vi "GetElements(Multiple).vi"(7 "Qualified Name":string, 8 "error in (no error)":errorcluster, 10 "keys":string[](array[string]), 11 "SMOConfigManagerCollection in":refnum<class "ConfigManagerCollection.lvclass">) -> (0 "error out":errorcluster, 1 "Found":bool[](array[boolean]), 2 "Values":string[](array[string]), 3 "SMOConfigManagerCollection out":refnum<class "ConfigManagerCollection.lvclass">)   [LabVIEW 2013, in "SMOConfig.lvlib" / "ConfigManagerCollection.lvclass"]
uses:
  ConfigManagerCollection.lvclass
  Manager/ConfigManager.lvclass
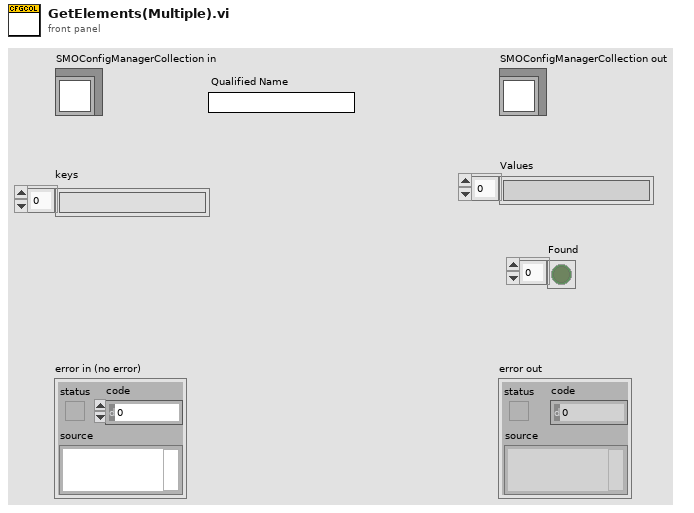
[diagram p1: front panel]
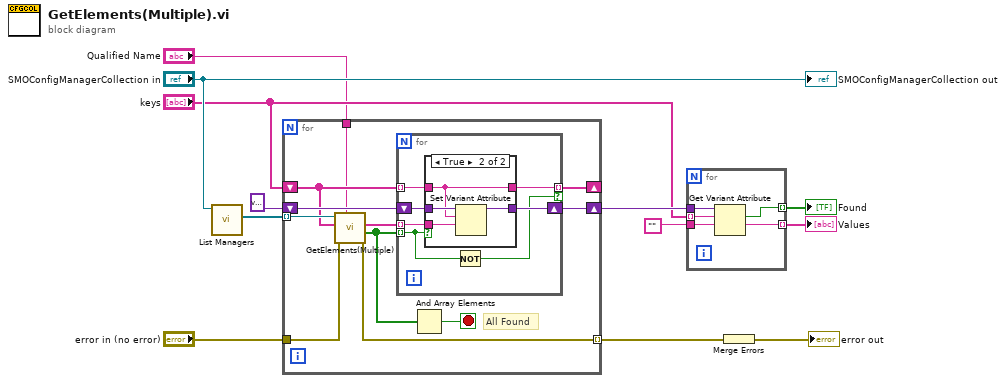
[diagram p0: block diagram]
diagram:
  n1 = call-dynamic "List Managers.vi"("SMOConfigManagerCollection in"="SMOConfigManagerCollection in") -> ("List"=w12:refnum<class "ConfigManager.lvclass">[])  [unwired: 9 in, 1 out]
  n2 = for {
    tunnel: w12 -> [w23] mode=indexing
    tunnel: "error in (no error)" -> [w21]
    tunnel: [w20] -> w11 mode=indexing
    shift-right: [w17] -> w6
    shift-left: variant ("variant") -> [w18]
    shift-right: [w14] -> _
    shift-left: "keys" -> [w15]
    tunnel: "Qualified Name" -> [w13]
    stop <- w22 stop-if-true
    # "All Found"
    n3 = call-dynamic "GetElements(Multiple).vi"("Qualified Name"=w13, "error in (no error)"=w21, "keys"=w15, "SMOConfigManager in"=w23) -> ("error out"=w20:errorcluster, "Found"=w19:bool[], "Values"=w16:string[])  [unwired: 4 in, 1 out]
    n4 = for {
      tunnel: w19 -> [w25] mode=indexing
      shift-right: [w30] -> w17
      shift-left: w18 -> [w29]
      tunnel: w15 -> [w28] mode=indexing
      tunnel: w16 -> [w27] mode=indexing
      tunnel: [w26] -> w14 mode=indexing if=w24
      n5 = case shown="True" w25 {
        tunnel: [w32 w34] -> w30
        tunnel: w29 -> [w32 w35]
        tunnel: w28 -> [w31 w33]
        tunnel: w27 -> [_ w36]
        tunnel: [w31 w33] -> w26
        frame False {
        }
        frame True {
          n6 = Set Variant Attribute(Variant=w35, name=w33, value=w36) -> (Variant out=w34:variant)  [unwired: 1 in, 2 out]
        }
      }
      n7 = Not(x=w25) -> (.not. x?=w24:bool)
    }
    n8 = And Array Elements(Boolean array=w19) -> (logical AND=w22:bool)
  }
  n9 = for {
    tunnel: w6 -> [w41]
    tunnel: "keys" -> [w40] mode=indexing
    tunnel: "" -> [w39]
    tunnel: [w38] -> w3 mode=indexing
    tunnel: [w37] -> w2 mode=indexing
    n10 = Get Variant Attribute(Variant=w41, name=w40, default value (empty Variant)=w39) -> (found=w37:bool, value=w38:string)  [unwired: 1 in, 2 out]
  }
  "Values" <- w3
  "Found" <- w2
  n11 = Merge Errors(w11) -> (→"error out":errorcluster)
  "SMOConfigManagerCollection out" <- "SMOConfigManagerCollection in"
